vi "Confidence Interval (Linear).vi"(0 "Y":dbl[](array[numeric]), 1 "confidence level":dbl=0.95 format="%.2f", 5 "X":dbl[](array[numeric]), 7 "Weight":dbl[](array[numeric]), 9 "slope":dbl, 11 "intercept":dbl) -> (4 "Upper Bound":dbl[](array[numeric]), 6 "Lower Bound":dbl[](array[numeric]), 8 "delta slope":dbl, 10 "delta intercept":dbl, 15 "error":i32)   [LabVIEW 2024, in "NI_AALPro.lvlib"]
doc: "<p>Calculates statistical intervals of the best linear fit for a data set (<strong>X</strong>, <strong>Y</strong>). You must <a href=\"nihelplauncher://docs/csh?context=lvcore_lvhowto_selectingdefaultinstpolyvi\">manually select the polymorphic instance</a> to use.</p>"
uses:
  NI_AALPro.lvlib
  <resource>/lvanlys.dll
panel:
  out "Coef. Upper Bound":dbl[](array[numeric])
  out "Coef. Lower Bound":dbl[](array[numeric])
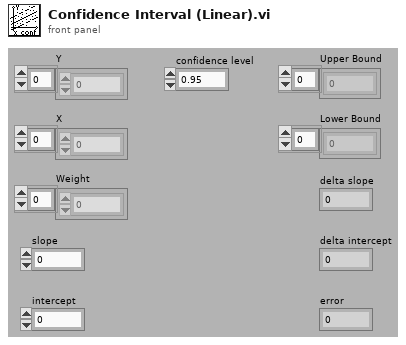
[diagram p1: front panel]
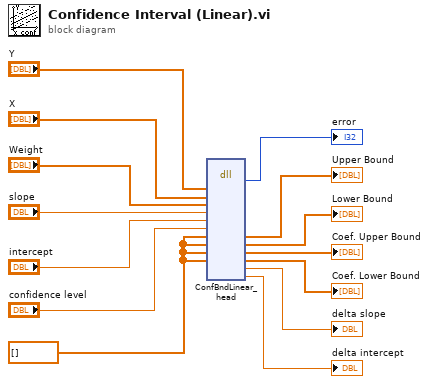
[diagram p0: block diagram]
diagram:
  w6 = dbl[] [] ("Best Linear Fit")
  n1 = dll-call lib="C:/Program Files (x86)/National Instruments/LabVIEW 2024/resource/lvanlys.*" fn="ConfBndLinear_head"("y"="Y", "x"="X", "weight"="Weight", "slope"="slope", "intercept"="intercept", "confidentLevel"="confidence level", "upper"=w6, "lower"=w6, "upperCoef"=w6, "lowerCoef"=w6) -> (→"error":i32, "upper"=→"Upper Bound":dbl[], "lower"=→"Lower Bound":dbl[], "upperCoef"=→"Coef. Upper Bound":dbl[], "lowerCoef"=→"Coef. Lower Bound":dbl[], "deltaSlope"=→"delta slope":dbl, "deltaIntcpt"=→"delta intercept":dbl)  [unwired: 11 in, 2 out]
